vi "CODMn启动流程.vi"() -> ()   [LabVIEW 2016]
uses:
  <vilib>/Utility/miscctls.llb/LVPointTypeDef.ctl
panel:
  out "加标回收实测值":sgl
  out "加标回收数据时间":timestamp
  out "跨度核查实测值":sgl
  out "跨度核查数据时间":timestamp
  out "空白实测值":sgl
  out "空白数据时间":timestamp
  out "水样实测值":sgl
  out "水样数据时间":timestamp
  out "启动记录":string
  out "流程运行中":bool
  out "启动次数":i32
  out "日期/时间":string
  out "运行状态":string
  out "步骤运行时间/秒":i32
  out "流程结束":bool
  out "当前步骤":T1(ring)
  in  "步骤时间/秒":T2={"步骤1时间"=2, "步骤2时间"=4, "步骤3时间"=5, "步骤4时间"=55, "步骤5时间"=30, "步骤6时间"=7, "步骤7时间"=0, "步骤8时间"=0, "步骤9时间"=0, "步骤10时间"=0}
  # "CODMn模块"
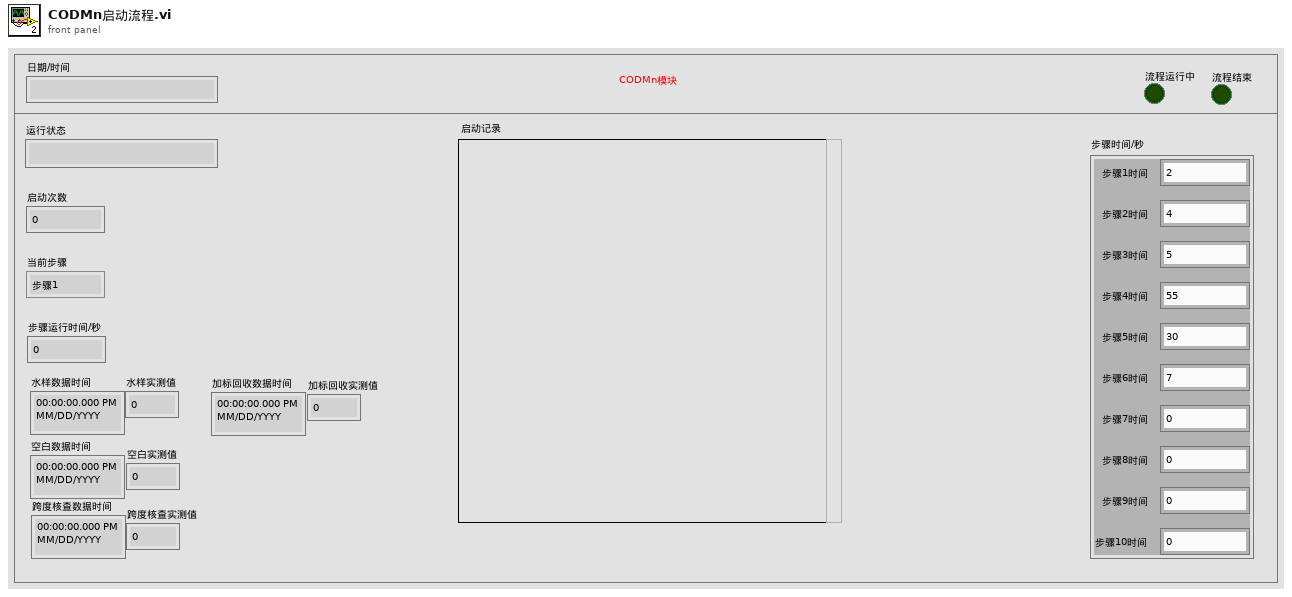
[diagram p1: front panel]
types:
  T1 = enum16{"步骤1", "步骤2", "步骤3", "步骤4", "步骤5", "步骤6", "步骤7", "步骤8", "步骤9", "步骤10"}
  T2 = cluster{"步骤1时间":i32, "步骤2时间":i32, "步骤3时间":i32, "步骤4时间":i32, "步骤5时间":i32, "步骤6时间":i32, "步骤7时间":i32, "步骤8时间":i32, "步骤9时间":i32, "步骤10时间":i32}
  T3 = enum16{"write register", "read register", "write and read register", "write coil", "read coil"}
  T4 = typedef "LVPointTypeDef.ctl" = cluster{"Horizontal":i16, "Vertical":i16}
  T5 = enum32{"Bad", "Idle", "Run top level", "Running"}
  T6 = cluster{"系统时间":timestamp, "工作状态":u16, "测量模式":u16, "告警代码":enum16{"无告警", "缺试剂告警", "缺水样告警", "缺蒸馏水告警", "缺标液告警", "仪表漏液告警", "标定异常告警", "超量程告警", "加热异常", "低试剂预警", "超上限告警", "超下限告警", "仪表内部其他异常", "滴定异常告警", "电极异常告警", "量程切换告警", "参数设置告警", "PH电极电位异常", "电导率电极异常", "浊度光度异常", "溶解氧电极异常", "溶解氧光强异常", "温度异常告警", "PH异常告警", "溶解氧异常告警", "电导率异常告警", "浊度异常告警", "叶绿素异常告警", "藻密度异常告警", "蓝绿藻异常告警", "ORP异常告警", "氨氮异常告警", "清洁刷异常告警", "SD卡异常告警", "蓝牙异常告警", "Wifi异常告警", "流程异常告警"}, "故障代码":enum16{"无故障", "电机故障", "温度故障", "通讯故障", "滴定故障"}, "日志代码":u16, "软件版本":u16, "F0":sgl, "F1":sgl, "F2":sgl, "F3":sgl, "T":sgl, "H":sgl, "id":u16, "flowid":u16, "量程":u16}
  T7 = cluster{"因子编码":u32, "单位":u16, "标样参考值":sgl, "水样数据时间":timestamp, "水样实测值":sgl, "水样数据标识":string, "标样数据时间":timestamp, "标样实测值":sgl, "标样数据标识":string, "空白数据时间":timestamp, "空白实测值":sgl, "空白数据标识":string, "零点核查数据时间":timestamp, "零点核查实测值":sgl, "零点核查数据标识":string, "跨度核查数据时间":timestamp, "跨度核查实测值":sgl, "跨度核查数据标识":string, "加标回收数据时间":timestamp, "加标回收实测值":sgl, "加标回收数据标识":string, "平行样数据时间":timestamp, "平行样实测值":sgl, "平行样数据标识":string}
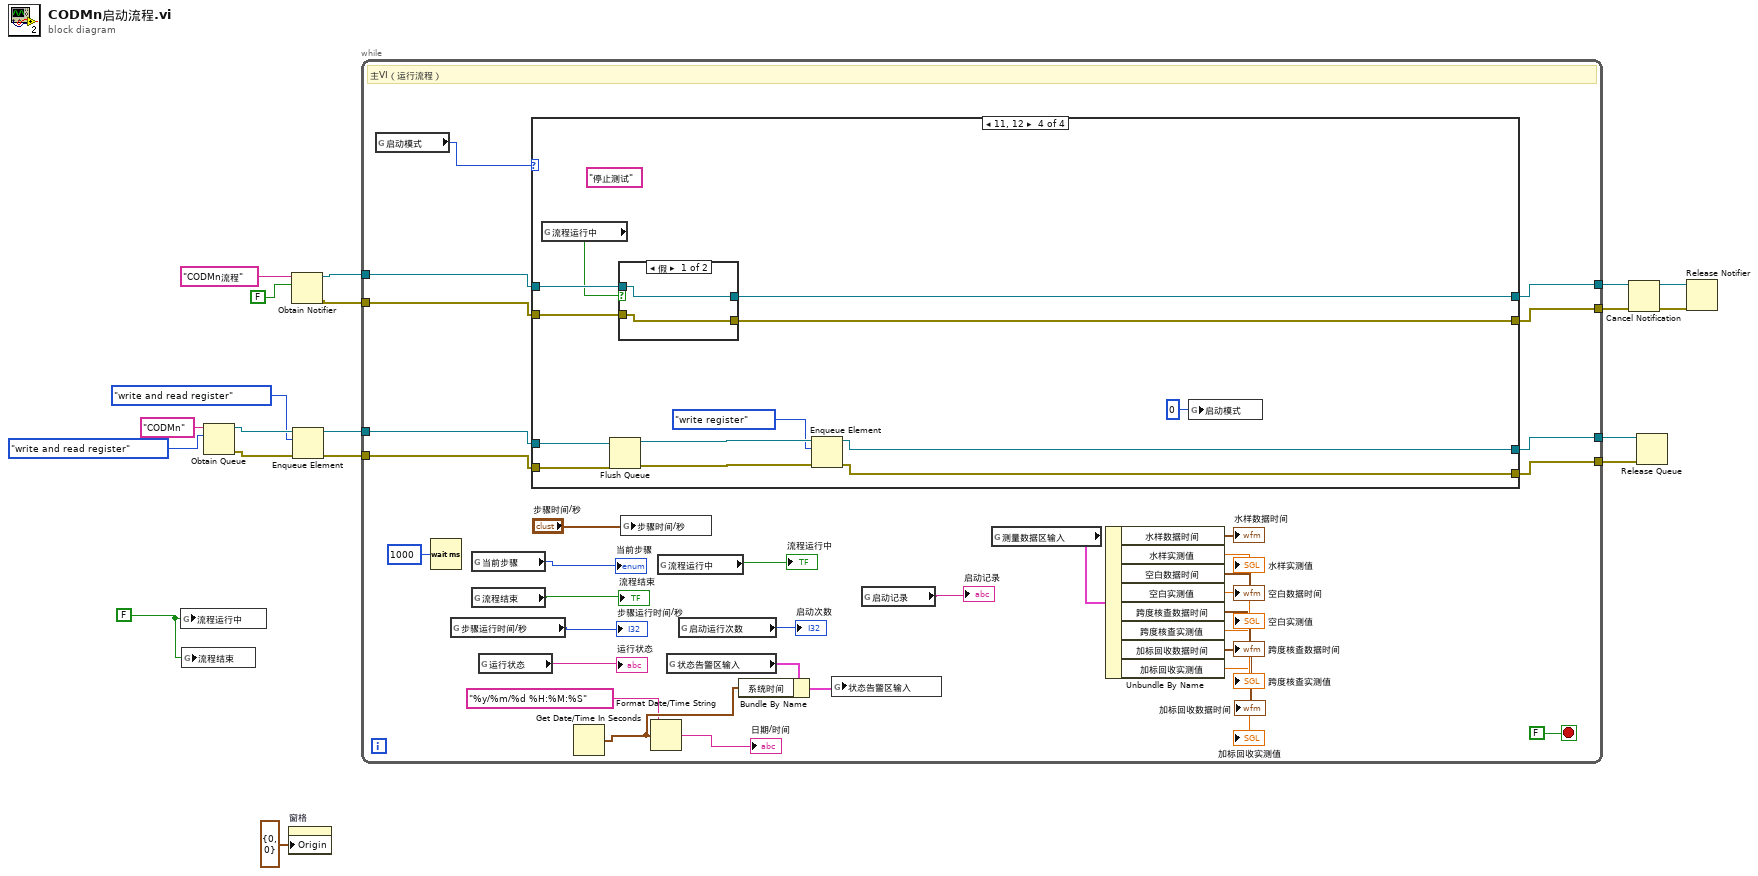
[diagram p0: block diagram]
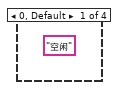
[diagram p2: hidden frame]
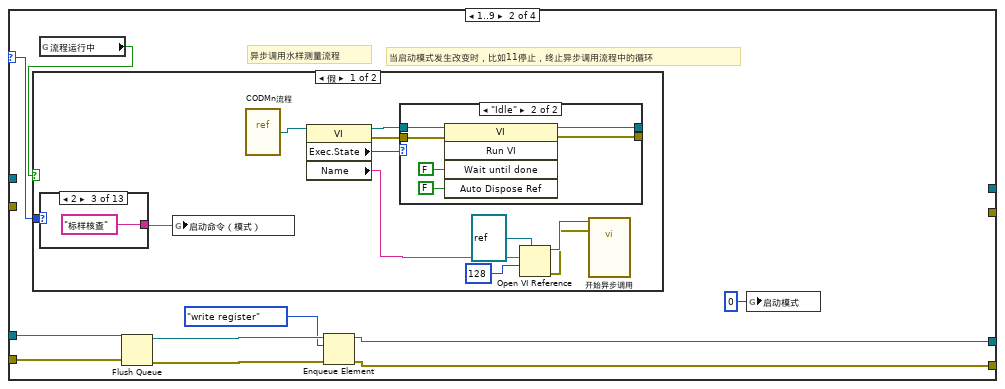
[diagram p3: hidden frame]
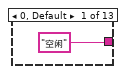
[diagram p5: hidden frame]
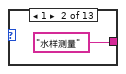
[diagram p6: hidden frame]
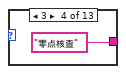
[diagram p7: hidden frame]
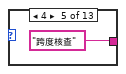
[diagram p8: hidden frame]
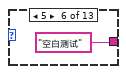
[diagram p9: hidden frame]
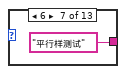
[diagram p10: hidden frame]
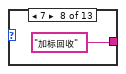
[diagram p11: hidden frame]
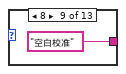
[diagram p12: hidden frame]
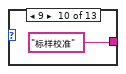
[diagram p13: hidden frame]
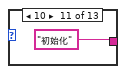
[diagram p14: hidden frame]
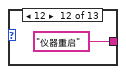
[diagram p15: hidden frame]
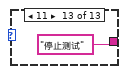
[diagram p16: hidden frame]
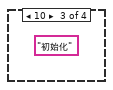
[diagram p18: hidden frame]
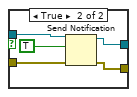
[diagram p19: hidden frame]
diagram:
  w10 = FALSE ("流程运行中")
  n1 = global write "CODMn全局.vi" "流程运行中"(w10) -> ()
  n2 = global write "CODMn全局.vi" "流程结束"(w10) -> ()
  n3 = Obtain Queue(name (unnamed)="CODMn" ("名称（未命名）"), element data type=T3."write and read register") -> (queue out=w7:refnum<queue>, error out=w6:errorcluster)  [unwired: 3 in, 1 out]
  n4 = property on="窗格" class="Pane"("Origin"=T4 {"Horizontal"=0, "Vertical"=0} ("原点")) -> ()  [unwired: 2 in, 2 out]
  n5 = Obtain Notifier(name (unnamed)="CODMn流程" ("名称（未命名）"), notification data type=FALSE) -> (notifier out=w15:refnum<notifier>, error out=w14:errorcluster)  [unwired: 2 in, 1 out]
  n6 = Enqueue Element(queue=w7, element=T3."write and read register", error in (no error)=w6) -> (queue out=w4:refnum<queue>, error out=w3:errorcluster)  [unwired: 1 in, 1 out]
  n7 = while {
    tunnel: w14 -> [w50]
    tunnel: w15 -> [w49]
    tunnel: [w48] -> w18
    tunnel: [w47] -> w19
    tunnel: w4 -> [w33]
    tunnel: w3 -> [w32]
    tunnel: [w31] -> w2
    tunnel: [w30] -> w1
    stop <- FALSE stop-if-true
    # "主VI（运行流程）"
    n8 = global read "CODMn全局.vi" "启动模式"() -> (w20:u16)
    n9 = Wait (ms)(milliseconds to wait=u32 1000 ("等待时间（毫秒）")) -> ()  [unwired: 1 out]
    n10 = global read "CODMn全局.vi" "步骤运行时间/秒"() -> (→"步骤运行时间/秒":i32)
    n11 = global read "CODMn全局.vi" "当前步骤"() -> (→"当前步骤":T1)
    n12 = global read "CODMn全局.vi" "流程结束"() -> (→"流程结束":bool)
    n13 = global read "CODMn全局.vi" "运行状态"() -> (→"运行状态":string)
    n14 = case shown="11, 12" w20 {
      selector: w20 -> [_ w62 _ _]
      tunnel: w50 -> [_ _ _ w107]
      tunnel: w49 -> [_ _ _ w106]
      tunnel: [_ _ _ w105] -> w48
      tunnel: [_ _ _ w104] -> w47
      tunnel: w33 -> [_ w58 _ w100]
      tunnel: w32 -> [_ w57 _ w99]
      tunnel: [_ w56 _ w98] -> w31
      tunnel: [_ w55 _ w97] -> w30
      frame 0, Default {
        (unwired) "空闲"
      }
      frame 1..9 {
        # "当启动模式发生改变时，比如11停止，终止异步调用流程中的循环"
        # "异步调用水样测量流程"
        n15 = global read "CODMn全局.vi" "流程运行中"() -> (w54:bool)
        n16 = case shown="假" w54 {
          tunnel: w62 -> [w64 _]
          frame False {
            n17 = case shown="2" w64 {
              tunnel: ["空闲" "水样测量" "标样核查" "零点核查" "跨度核查" "空白测试" "平行样测试" "加标回收" "空白校准" "标样校准" "初始化" "仪器重启" "停止测试"] -> w63
              frame 0, Default {
              }
              frame 1 {
              }
              frame 2 {
              }
              frame 3 {
              }
              frame 4 {
              }
              frame 5 {
              }
              frame 6 {
              }
              frame 7 {
              }
              frame 8 {
              }
              frame 9 {
              }
              frame 10 {
              }
              frame 12 {
              }
              frame 11 {
              }
            }
            n18 = global write "CODMn全局.vi" "启动命令（模式）"(w63) -> ()
            n19 = vi-ref "CODMn流程.vi"() -> (w73:refnum<vi>)
            n20 = property class="VI"(reference=w73) -> (reference out=w72:refnum<vi>, error out=w70:errorcluster, "Exec.State"=w71:T5, "Name"=w65:string)  [unwired: 1 in]
            n21 = case shown="\"Idle\"" w71 {
              tunnel: w72 -> [w75 w81]
              tunnel: [w75 w80] -> _
              tunnel: w70 -> [w74 w77]
              tunnel: [w74 w76] -> _
              frame "Bad", Default {
              }
              frame "Idle" {
                n22 = invoke class="VI" method="Run VI"(reference=w81, error in=w77, "Wait until done"=FALSE ("结束前等待"), "Auto Dispose Ref"=FALSE ("自动销毁引用")) -> (reference out=w80:refnum<vi>, error out=w76:errorcluster)  [unwired: 1 in, 3 out]
              }
            }
            n23 = Open VI Reference(type specifier VI Refnum (for type only)=refnum<vi> refnum ("类型说明符VI引用句柄（仅用于类型）"), vi path=w65, options=128 ("选项")) -> (vi reference=w69:refnum<vi>, error out=w67:errorcluster)  [unwired: 3 in]
            n24 = call-by-ref "开始异步调用"(reference=w69, error in=w67) -> ()  [unwired: 12 in, 2 out]
          }
          frame True {
          }
        }
        n25 = Flush Queue(queue=w58, error in (no error)=w57) -> (queue out=w61:refnum<queue>, error out=w60:errorcluster)  [unwired: 1 out]
        n26 = Enqueue Element(queue=w61, element=T3."write register", error in (no error)=w60) -> (queue out=w56:refnum<queue>, error out=w55:errorcluster)  [unwired: 1 in, 1 out]
        n27 = global write "CODMn全局.vi" "启动模式"(u16 0 ("启动模式")) -> ()
      }
      frame 10 {
        (unwired) "初始化"
      }
      frame 11, 12 {
        (unwired) "停止测试"
        n28 = global read "CODMn全局.vi" "流程运行中"() -> (w96:bool)
        n29 = Flush Queue(queue=w100, error in (no error)=w99) -> (queue out=w103:refnum<queue>, error out=w102:errorcluster)  [unwired: 1 out]
        n30 = case shown="假" w96 {
          tunnel: w107 -> [w108 w113]
          tunnel: w106 -> [w109 w112]
          tunnel: [w109 w111] -> w105
          tunnel: [w108 w110] -> w104
          frame False {
          }
          frame True {
            n31 = Send Notification(notification=TRUE ("通知"), notifier=w112, error in (no error)=w113) -> (notifier out=w111:refnum<notifier>, error out=w110:errorcluster)
          }
        }
        n32 = Enqueue Element(queue=w103, element=T3."write register", error in (no error)=w102) -> (queue out=w98:refnum<queue>, error out=w97:errorcluster)  [unwired: 1 in, 1 out]
        n33 = global write "CODMn全局.vi" "启动模式"(u16 0 ("启动模式")) -> ()
      }
    }
    n34 = Get Date/Time In Seconds() -> (seconds since 1Jan1904=w46:timestamp)
    n35 = global write "CODMn全局.vi" "步骤时间/秒"("步骤时间/秒") -> ()
    n36 = Format Date/Time String(time format string (%c)="%y/%m/%d %H:%M:%S" ("时间格式字符串(%c)"), seconds (now)=w46) -> (date/time string=→"日期/时间":string)  [unwired: 1 in]
    n37 = global read "CODMn全局.vi" "流程运行中"() -> (→"流程运行中":bool)
    n38 = global read "CODMn全局.vi" "状态告警区输入"() -> (w43:T6)
    n39 = global read "CODMn全局.vi" "启动运行次数"() -> (→"启动次数":i32)
    n40 = Bundle By Name(cluster=w43, "系统时间"=w46) -> (w42:T6)
    n41 = global write "CODMn全局.vi" "状态告警区输入"(w42) -> ()
    n42 = global read "CODMn全局.vi" "启动记录"() -> (→"启动记录":string)
    n43 = global read "CODMn全局.vi" "测量数据区输入"() -> (w29:T7)
    n44 = Unbundle By Name(w29) -> ("水样数据时间"=→"水样数据时间":timestamp, "水样实测值"=→"水样实测值":sgl, "空白数据时间"=→"空白数据时间":timestamp, "空白实测值"=→"空白实测值":sgl, "跨度核查数据时间"=→"跨度核查数据时间":timestamp, "跨度核查实测值"=→"跨度核查实测值":sgl, "加标回收数据时间"=→"加标回收数据时间":timestamp, "加标回收实测值"=→"加标回收实测值":sgl)
  }
  n45 = Cancel Notification(0:w18, 3:w19) -> (8:w17:refnum<notifier>, 11:w16:errorcluster)  [unwired: 1 out]
  n46 = Release Queue(queue=w2, error in (no error)=w1) -> ()  [unwired: 1 in, 3 out]
  n47 = Release Notifier(notifier=w17, error in (no error)=w16) -> ()  [unwired: 1 in, 3 out]
